vi "create daemon.vi"(8 "error in (no error)":errorcluster) -> (0 "error out":errorcluster)   [LabVIEW 2016, in "数据传输系统-06.lvlib" / "update.lvlib"]
uses:
  update.lvlib
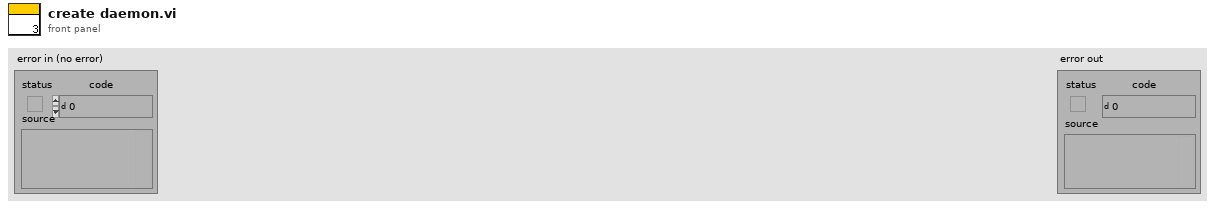
[diagram p1: front panel]
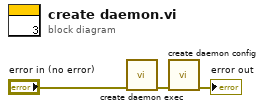
[diagram p0: block diagram]
diagram:
  n1 = call "create daemon exec.vi"("error in (no error)"="error in (no error)") -> ("error out"=w3:errorcluster)  [unwired: 10 in]
  n2 = call "create daemon config.vi"("error in (no error)"=w3) -> ("error out"=→"error out":errorcluster)  [unwired: 10 in]
